vi "Get UDV Data.vi"(7 "Channel Type":T1, 8 "error in (no error)":errorcluster, 11 "Channel Ref List in":T2[](array[typedef]) format="%.0x") -> (0 "error out":errorcluster, 2 "UDV Data":T3[](array[typedef]) {"VS ref" format="%.0x"}, 3 "Channel Ref List out":T2[](array[typedef]) format="%.0x")   [LabVIEW 2011, in "Scan Engine Custom Device.lvlib"]
uses:
  Scan Engine Custom Device.lvlib
  Type Defs/UDV Data.ctl
  <vilib>/NI Veristand/Custom Device API/Custom Device Item Ref.ctl
  Type Defs/UDV Data Type.ctl
  Type Defs/FXP Config.ctl
  <vilib>/NI Veristand/Custom Device API/Custom Device Channel Type.ctl
  Globals/Scan Engine GUIDs.vi
  Globals/Property Strings.vi
  <vilib>/NI Veristand/Custom Device API/Get Item Property (String).vi
  <vilib>/NI Veristand/Custom Device API/Get Item Property (U16).vi
  <vilib>/NI Veristand/Custom Device API/Get Item Property (Variant).vi
  <vilib>/NI Veristand/Custom Device API/Custom Device API.lvlib
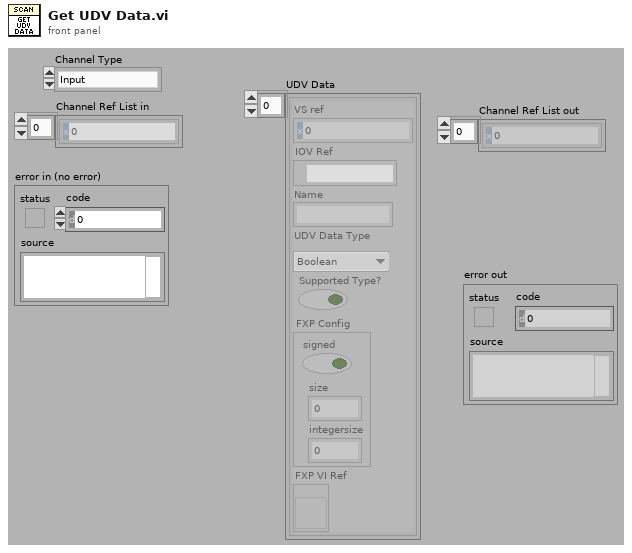
[diagram p1: front panel]
types:
  T1 = typedef "Custom Device API.lvlib/Custom Device Channel Type.ctl" = enum16{"Input", "Output"}
  T2 = typedef "Custom Device API.lvlib/Custom Device Item Ref.ctl" = u64
  T3 = typedef "Scan Engine Custom Device.lvlib/UDV Data.ctl" = cluster{"VS ref":T2, "IOV Ref":refnum<k21>, "Name":string, "UDV Data Type":T4, "Supported Type?":bool, "FXP Config":T5, "FXP VI Ref":refnum<vi>}
  T4 = typedef "Scan Engine Custom Device.lvlib/UDV Data Type.ctl" = enum16{"Boolean", "Fixed Point", "Int8", "Int16", "Int32", "Int64", "U32 Bit Field", "UInt8", "UInt16", "UInt32", "UInt64", "Other"}
  T5 = typedef "Scan Engine Custom Device.lvlib/FXP Config.ctl" = cluster{"signed":bool, "size":u32, "integersize":i32}
  T6 = typedef "Custom Device API.lvlib/Custom Device Item Info.ctl" = cluster{"Name":string, "Is Channel":bool, "GUID":string}
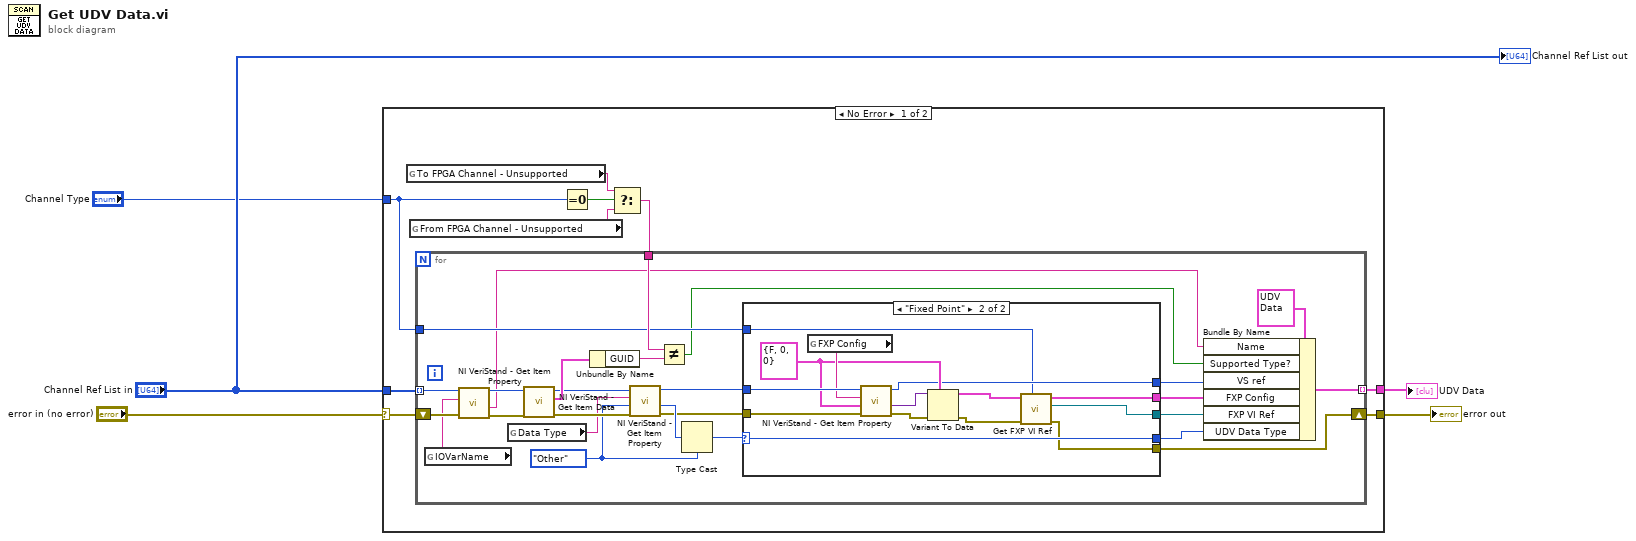
[diagram p0: block diagram]
diagram:
  n1 = case shown="No Error" "error in (no error)" {
    selector: "error in (no error)" -> [w11 w58]
    tunnel: [w14 _] -> w5
    tunnel: "Channel Ref List in" -> [w13 _]
    tunnel: [w12 w58] -> w3
    tunnel: "Channel Type" -> [w6 _]
    frame No Error {
      n2 = global read "Scan Engine GUIDs.vi" "To FPGA Channel - Unsupported"() -> (w9:string)
      n3 = global read "Scan Engine GUIDs.vi" "From FPGA Channel - Unsupported"() -> (w8:string)
      n4 = Equal To 0?(x=w6) -> (x = 0?=w10:bool)
      n5 = Select(t=w9, s=w10, f=w8) -> (s? t:f=w7:string)
      n6 = for {
        tunnel: w13 -> [w17] mode=indexing
        shift-right: [w26] -> w12
        shift-left: w11 -> [w20]
        tunnel: [w25] -> w14 mode=indexing
        tunnel: w7 -> [w24]
        tunnel: w6 -> [w23]
        w34 = UDV_Data_Type."Other" ("UDV Data Type out")
        n7 = global read "Property Strings.vi" "IOVarName"() -> (w16:string)
        n8 = call-poly <vilib>:"NI VeriStand - Get Item Property.vi"("error in (no error)"=w20, "Property Name"=w16, "Item Ref in"=w17) -> ("error out"=w19:errorcluster, "Value"=w15:string, "Item Ref out"=w18:T2)  [unwired: 5 in, 1 out]
        n9 = global read "Property Strings.vi" "Data Type"() -> (w35:string)
        n10 = call <vilib>:"NI VeriStand - Get Item Data.vi"("error in (no error)"=w19, "Item Ref in"=w18) -> ("error out"=w36:errorcluster, "Item Info"=w40:T6, "Item Ref out"=w37:T2)  [unwired: 7 out]
        n11 = Unbundle By Name(w40) -> ("GUID"=w39:string)
        n12 = call-poly <vilib>:"NI VeriStand - Get Item Property.vi"("error in (no error)"=w36, "Default Value"=w34, "Property Name"=w35, "Item Ref in"=w37) -> ("error out"=w31:errorcluster, "Value"=w33:u16, "Item Ref out"=w30:T2)  [unwired: 4 in, 1 out]
        n13 = Not Equal?(x=w24, y=w39) -> (x != y?=w22:bool)
        n14 = Type Cast(type=w34, x=w33) -> (*(type *) &x=w32:T4)
        n15 = case shown="\"Fixed Point\"" w32 {
          selector: w32 -> [w43 w50]
          tunnel: w31 -> [w41 w56]
          tunnel: w30 -> [w42 w57]
          tunnel: [_ w48] -> w29
          tunnel: [w42 w51] -> w28
          tunnel: [w43 w50] -> w27
          tunnel: [w41 w46] -> w26
          tunnel: w23 -> [_ w45]
          tunnel: [_ w44] -> w21
          frame Default {
          }
          frame "Fixed Point" {
            w52 = T5 {"signed"=FALSE, "size"=0, "integersize"=0} ("FXP Config")
            n16 = global read "Property Strings.vi" "FXP Config"() -> (w55:string)
            n17 = call-poly <vilib>:"NI VeriStand - Get Item Property.vi"("error in (no error)"=w56, "Default Value"=w52, "Property Name"=w55, "Item Ref in"=w57) -> ("error out"=w54:errorcluster, "Value"=w53:variant, "Item Ref out"=w51:T2)  [unwired: 4 in, 1 out]
            n18 = Variant To Data(error in=w54, type=w52, Variant=w53) -> (data=w49:T5, error out=w47:errorcluster)
            n19 = call "Get FXP VI Ref.vi"("Channel Type"=w45, "error in (no error)"=w47, "FXP Config in"=w49) -> ("error out"=w46:errorcluster, "FXP VI Ref"=w44:refnum<vi>, "FXP Config out"=w48:T5)  [unwired: 6 in]
          }
        }
        n20 = Bundle By Name(cluster=T3 {"VS ref"=0, "IOV Ref"="", "Name"="", "UDV Data Type"=enum."Boolean", "Supported Type?"=FALSE, "FXP Config"={"signed"=FALSE, "size"=0, "integersize"=0}, "FXP VI Ref"=refnum} ("UDV Data"), "Name"=w15, "Supported Type?"=w22, "VS ref"=w28, "FXP Config"=w29, "FXP VI Ref"=w21, "UDV Data Type"=w27) -> (w25:T3)
      }
    }
    frame Error {
    }
  }
  "UDV Data" <- w5
  "error out" <- w3
  "Channel Ref List out" <- "Channel Ref List in"
